vi "DisplayPanel.vi"() -> ()   [LabVIEW 2013]
uses:
  MvLVLib/MvCameraControl.lvlib
  <vilib>/picture/picture.llb/imagedata.ctl
panel:
  out "GenTLDevInfoArray":T1(array[cluster])
  out "GenTLIfInfoArray":T2(array[cluster])
  in  "Refresh Interaces":bool
  in  "Interface List":u16(ring)
  in  "pConvertInfo In":T3
  out "PixelFormat":u32
  out "handle out":u64
  in  "handle":u64
  in  "Rectangle":T4
  in  "image data":T5 caption="图像数据"
  out "Picture":picture
  out "PayloadSize":u32
  out "pFrameInfoEx out":T6
  out "nHeight":u32
  out "nWidth":u32
  out "Acquisision Flag":bool
  in  "Trigger Mode":bool
  in  "Continuous":bool
  out "打开标志":bool
  in  "stop":bool
  in  "Trigger Once":bool
  in  "Stop":bool
  in  "Start":bool
  in  "Open Device":bool
  in  "Close Device":bool
  in  "error in (no error) 2":errorcluster caption="错误输入（无错误）"
  in  "Refresh Devices":bool
  in  "Device List":u16(ring)
  # "Initialize"
  # "Acquisition"
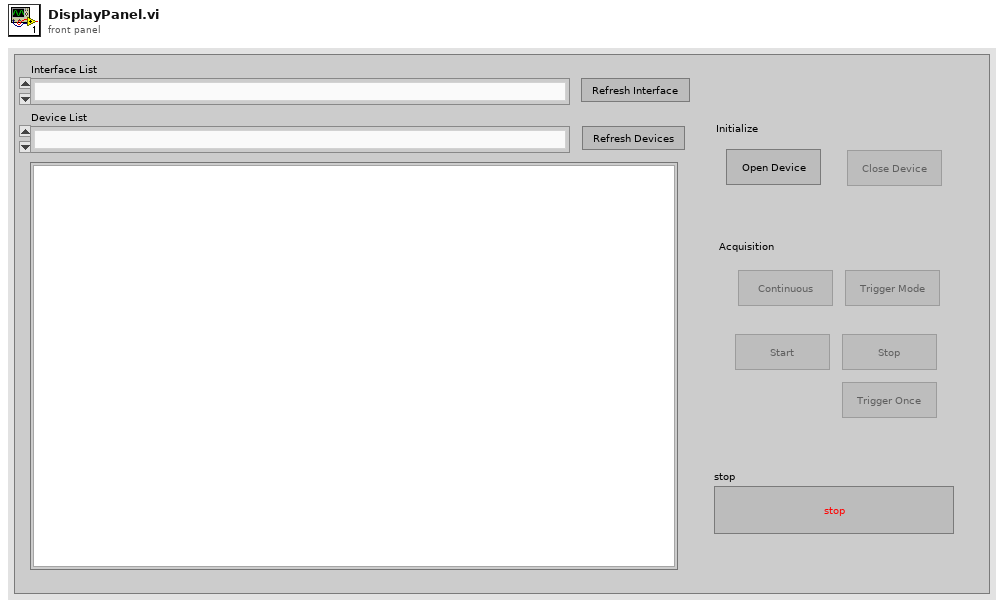
[diagram p1: front panel]
types:
  T1 = cluster{"chInterfaceID":string, "chDeviceID":string, "chVendorName":string, "chModelName":string, "chTLType":string, "chDisplayName":string, "chUserDefinedName":string, "chSerialNumber":string, "chDeviceVersion":string, "nCtiIndex":u32, "nReserved[0]":u32, "nReserved[1]":u32, "nReserved[2]":u32, "nReserved[3]":u32, "nReserved[4]":u32, "nReserved[5]":u32, "nReserved[6]":u32, "nReserved[7]":u32}[]
  T2 = cluster{"chInterfaceID":string, "chTLType":string, "chDisplayName":string, "nCtiIndex":u32, "nReserved[0]":u32, "nReserved[1]":u32, "nReserved[2]":u32, "nReserved[3]":u32, "nReserved[4]":u32, "nReserved[5]":u32, "nReserved[6]":u32, "nReserved[7]":u32}[]
  T3 = cluster{"nWidth":u16, "nHeight":u16, "enSrcPixelType":u32, "nSrcDataLen":u32, "enDstPixelType":u32, "nDstLen":u32, "nDstBufferSize":u32, "nRes0":u32, "nRes1":u32, "nRes2":u32, "nRes3":u32}
  T4 = cluster{"left":i16, "top":i16, "right":i16, "bottom":i16}
  T5 = typedef "imagedata.ctl" = cluster{"image type":i32, "image depth":i32, "image":u8[], "mask":u8[], "colors":u32[], "Rectangle":cluster{"left":i16, "top":i16, "right":i16, "bottom":i16}}
  T6 = cluster{"nWidth":u16, "nHeight":u16, "enPixelType":i32, "nFrameNum":u32, "nDevTimeStampHigh":u32, "nDevTimeStampLow":u32, "nReserved0":u32, "nHostTimeStamp":i64, "nFrameLen":u32, "nSecondCount]":u32, "nCycleCount":u32, "nCycleOffset":u32, "fGain":u32, "fExposureTime":u32, "nAverageBrightness":u32, "nRed":u32, "nGreen":u32, "nBlue":u32, "nFrameCounter":u32, "nTriggerIndex":u32, "nInput":u32, "nOutput":u32, "nOffsetX":u32, "nOffsetY":u32, "nReserved[0]":u32, "nReserved[1]":u32, "nReserved[2]":u32, "nReserved[3]":u32, "nReserved[4]":u32, "nReserved[5]":u32, "nReserved[6]":u32, "nReserved[7]":u32, "nReserved[8]":u32, "nReserved[9]":u32, "nReserved[10]":u32, "nReserved[11]":u32, "nReserved[12]":u32, "nReserved[13]":u32, "nReserved[14] 10":u32, "nReserved[15] 11":u32, "nReserved[16] 12":u32, "nReserved[17] 13":u32, "nReserved[18] 14":u32, "nReserved[19] 15":u32, "nReserved[20] 16":u32, "nReserved[21] 17":u32, "nReserved[22] 18":u32, "nReserved[23] 19":u32, "nReserved[24] 20":u32, "nReserved[25] 21":u32, "nReserved[26] 22":u32, "nReserved[27] 23":u32, "nReserved[28] 24":u32, "nReserved[29] 25":u32, "nReserved[30] 26":u32, "nReserved[31] 27":u32, "nReserved[32] 28":u32, "nReserved[33] 29":u32, "nReserved[34] 30":u32, "nReserved[35] 31":u32, "nReserved[36] 32":u32, "nReserved[37] 33":u32, "nReserved[38] 34":u32, "nReserved[39] 35":u32, "nReserved[40] 36":u32}
  T7 = enum8{"Enabled", "Disabled", "Disabled and Grayed Out"}
  T8 = cluster{"nCurValue":u32, "nMax":u32, "nMin":u32, "nInc":u32, "nReserved[0]":u32, "nReserved[1]":u32, "nReserved[2]":u32, "nReserved[3]":u32}
  T9 = cluster{"nCurValue":u32, "nSupportedNum":u32, "nSupportValue":u32[], "nReserved[0]":u32, "nReserved[1]":u32, "nReserved[2]":u32, "nReserved[3]":u32}
  T10 = cluster{"chInterfaceID":string, "chTLType":string, "chDisplayName":string, "nCtiIndex":u32, "nReserved[0]":u32, "nReserved[1]":u32, "nReserved[2]":u32, "nReserved[3]":u32, "nReserved[4]":u32, "nReserved[5]":u32, "nReserved[6]":u32, "nReserved[7]":u32}
  T11 = cluster{"nWidth":u32, "nHeight":u32, "enSrcPixelType":u32, "nSrcDataLen":u32, "enDstPixelType":u32, "nDstLen":u32, "nDstBufferSize":u32, "nRes0":u32, "nRes1":u32, "nRes2":u32, "nRes3":u32}
  T12 = cluster{"chInterfaceID":string, "chDeviceID":string, "chVendorName":string, "chModelName":string, "chTLType":string, "chDisplayName":string, "chUserDefinedName":string, "chSerialNumber":string, "chDeviceVersion":string, "nCtiIndex":u32, "nReserved[0]":u32, "nReserved[1]":u32, "nReserved[2]":u32, "nReserved[3]":u32, "nReserved[4]":u32, "nReserved[5]":u32, "nReserved[6]":u32, "nReserved[7]":u32}
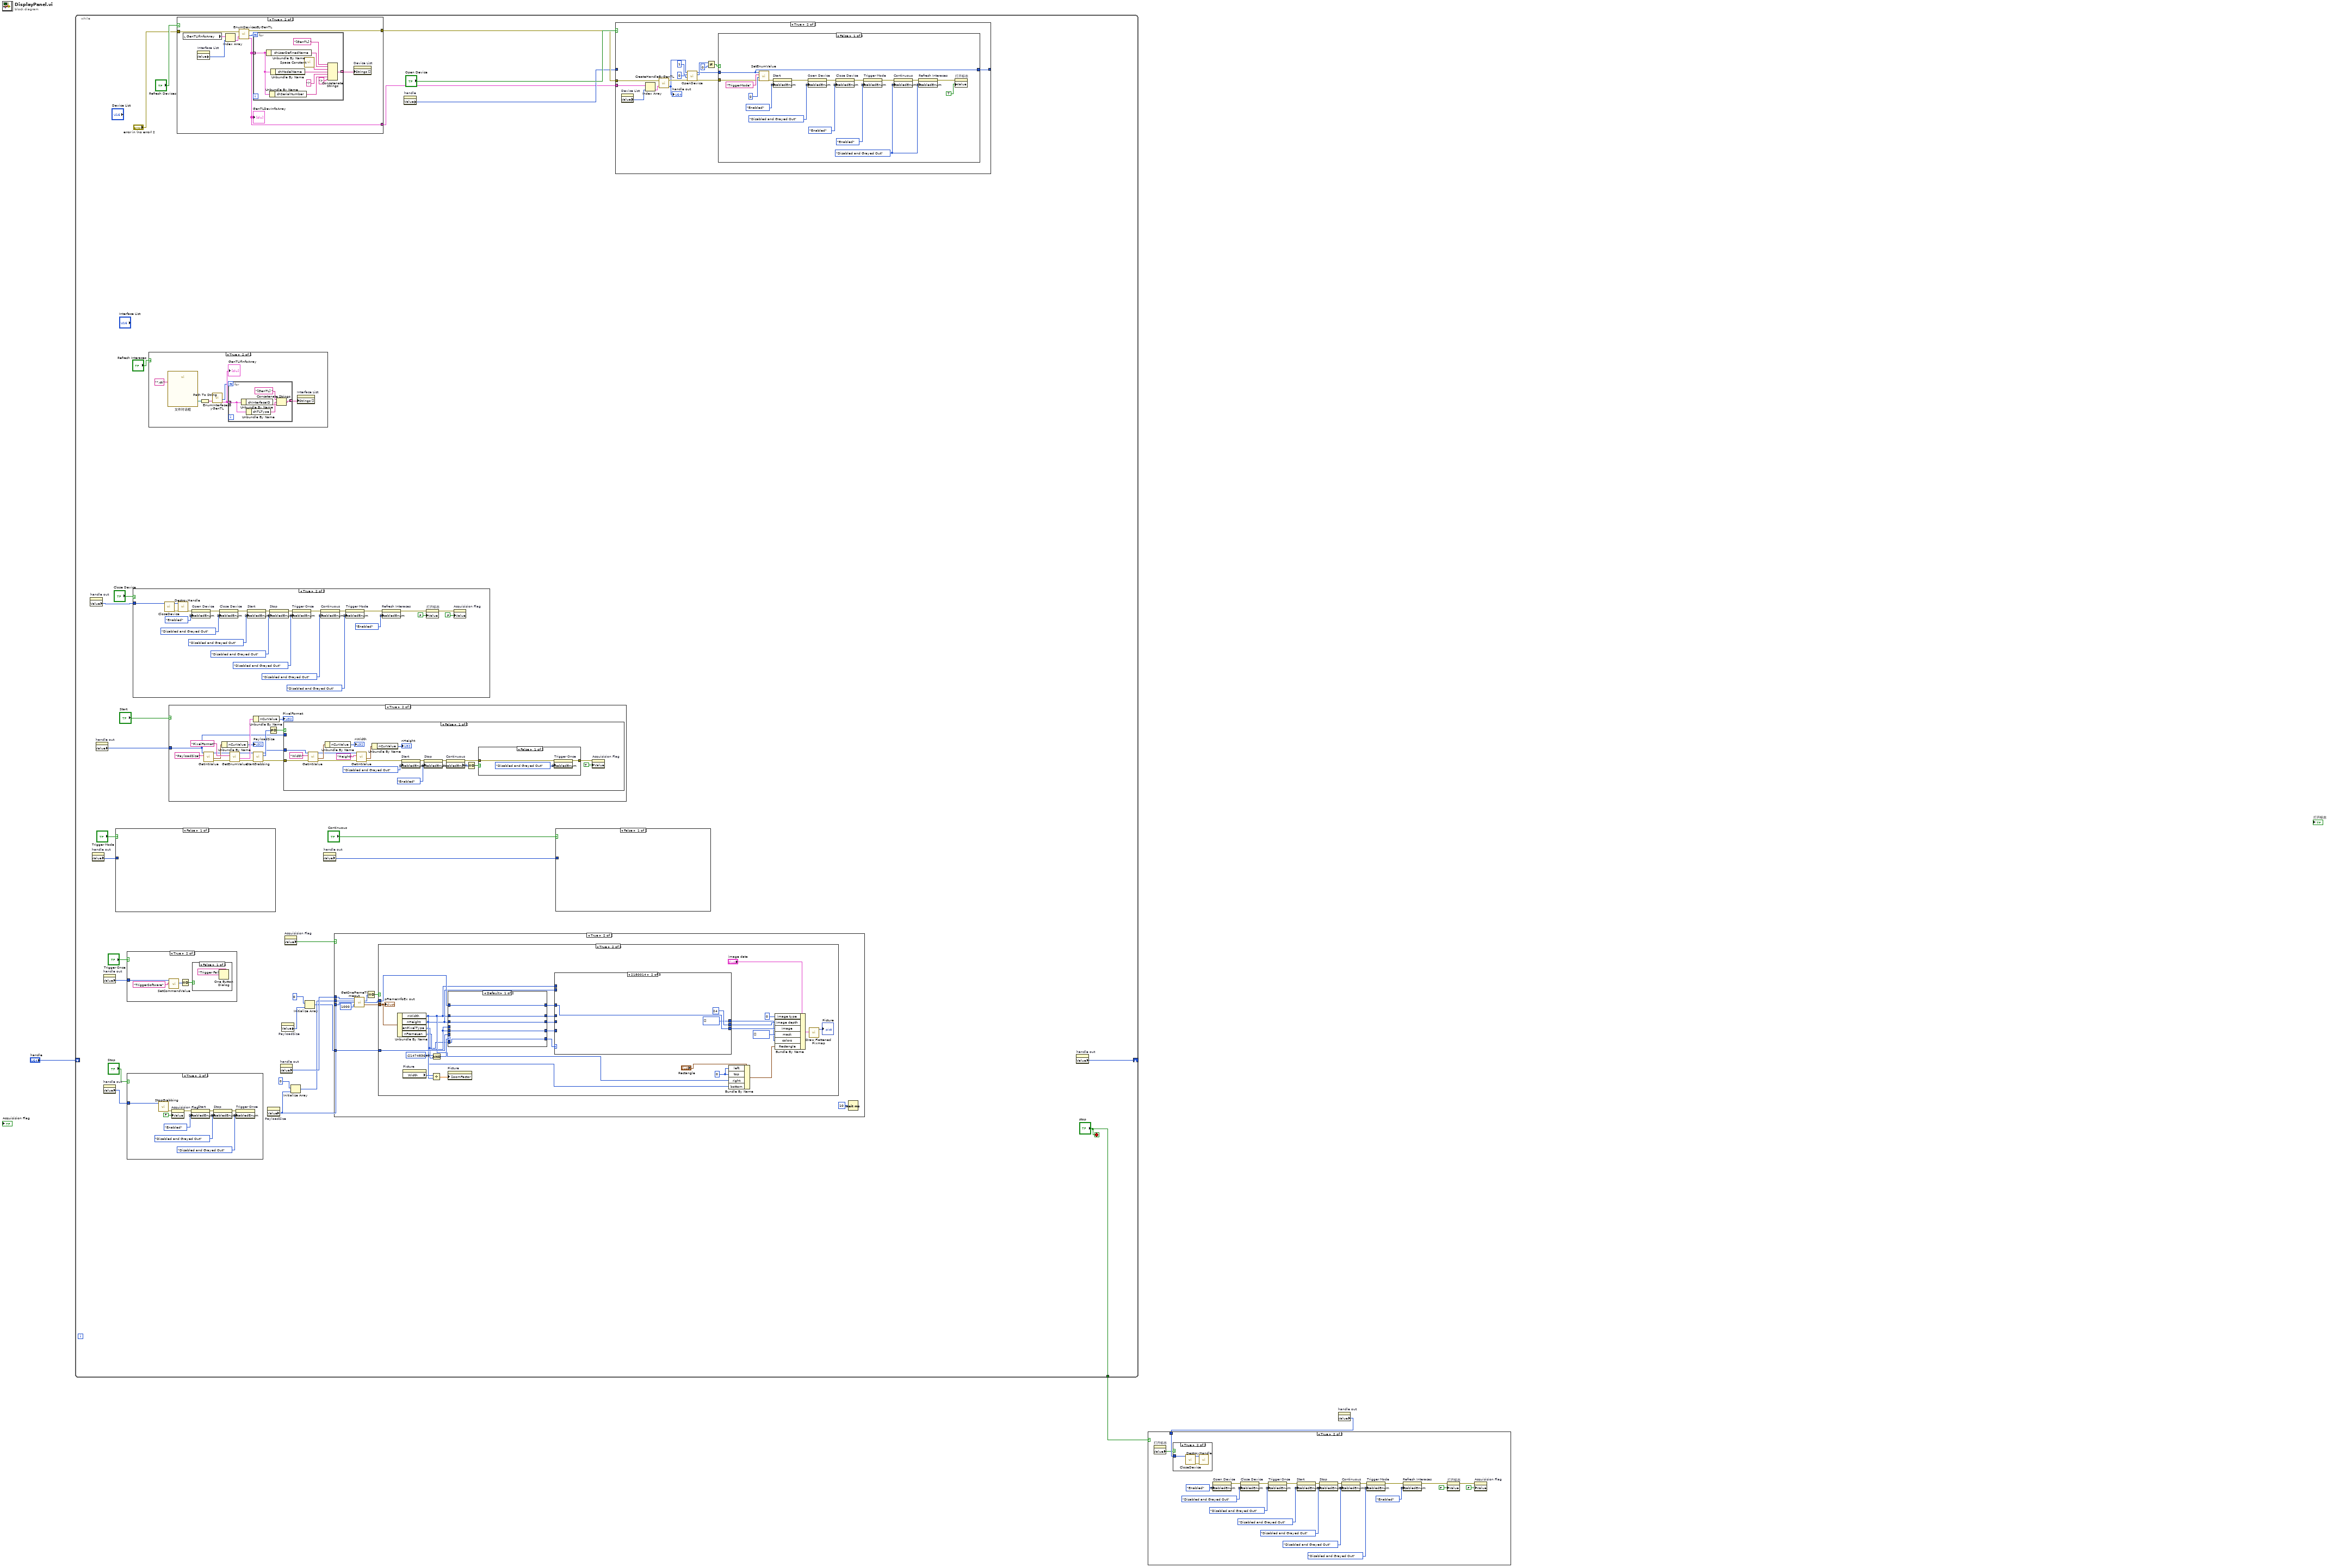
[diagram p0: block diagram]
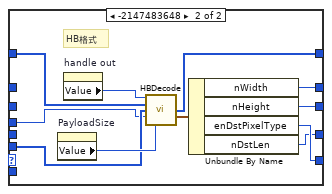
[diagram p7: hidden frame]
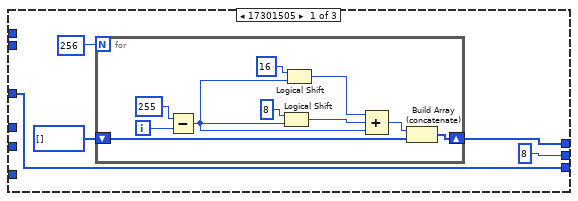
[diagram p8: hidden frame]
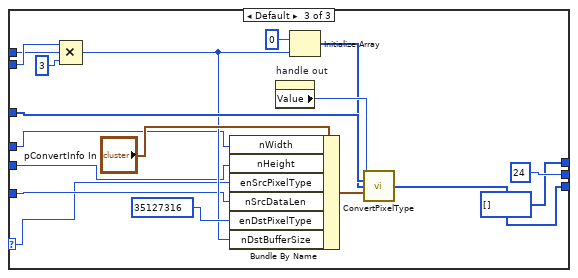
[diagram p9: hidden frame]
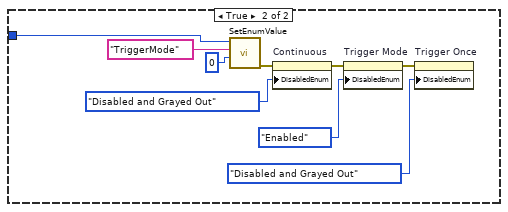
[diagram p11: hidden frame]
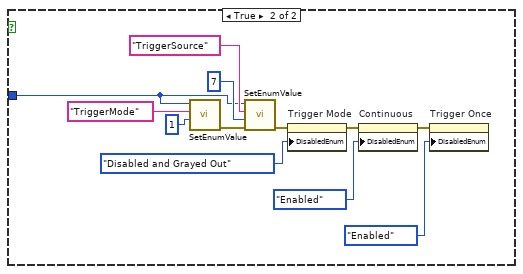
[diagram p12: hidden frame]
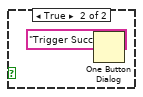
[diagram p14: hidden frame]
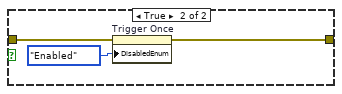
[diagram p16: hidden frame]
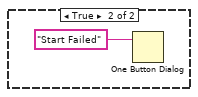
[diagram p17: hidden frame]
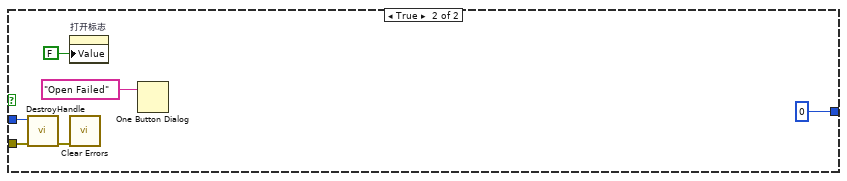
[diagram p20: hidden frame]
diagram:
  n1 = while {
    tunnel: ["stop"] -> w3
    shift-right: [w20] -> _
    shift-left: "handle" -> [_]
    stop <- "stop" stop-if-true
    n2 = property on="handle out" class="DigNum (strict)"() -> ("Value"=w18:u64)  [unwired: 2 in, 2 out]
    n3 = property on="handle out" class="DigNum (strict)"() -> ("Value"=w13:u64)  [unwired: 2 in, 2 out]
    n4 = property on="handle out" class="DigNum (strict)"() -> ("Value"=w14:u64)  [unwired: 2 in, 2 out]
    n5 = property on="handle out" class="DigNum (strict)"() -> ("Value"=w17:u64)  [unwired: 2 in, 2 out]
    n6 = property on="handle out" class="DigNum (strict)"() -> ("Value"=w16:u64)  [unwired: 2 in, 2 out]
    n7 = case shown="False" "Trigger Mode" {
      tunnel: w13 -> [_ w151]
      frame False {
      }
      frame True {
        n8 = call "SetEnumValue.vi"("nValue"=u32 1, "strKey"="TriggerMode", "handle"=w151) -> ("error out"=w157:errorcluster)  [unwired: 6 in, 2 out]
        n9 = call "SetEnumValue.vi"("error in (no error)"=w157, "nValue"=u32 7, "strKey"="TriggerSource", "handle"=w151) -> ("error out"=w156:errorcluster)  [unwired: 5 in, 2 out]
        n10 = property on="Trigger Mode" class="Bool"(error in=w156, "DisabledEnum"=T7."Disabled and Grayed Out" ("禁用")) -> (error out=w155:errorcluster)  [unwired: 1 in, 1 out]
        n11 = property on="Continuous" class="Bool"(error in=w155, "DisabledEnum"=T7."Enabled" ("禁用")) -> (error out=w153:errorcluster)  [unwired: 1 in, 1 out]
        n12 = property on="Trigger Once" class="Bool"(error in=w153, "DisabledEnum"=T7."Enabled" ("禁用")) -> ()  [unwired: 1 in, 2 out]
      }
    }
    n13 = case shown="True" "Trigger Once" {
      tunnel: w17 -> [_ w166]
      frame False {
      }
      frame True {
        n14 = call "SetCommandValue.vi"("strValue"="TriggerSoftware", "handle"=w166) -> ("function return"=w164:i32)  [unwired: 7 in, 2 out]
        n15 = Equal To 0?(x=w164) -> (x = 0?=w163:bool)
        n16 = case shown="False" w163 {
          frame False {
            n17 = One Button Dialog(message="Trigger Failed") -> ()  [unwired: 1 in, 1 out]
          }
          frame True {
            n18 = One Button Dialog(message="Trigger Success") -> ()  [unwired: 1 in, 1 out]
          }
        }
      }
    }
    n19 = case shown="True" "Stop" {
      tunnel: w16 -> [_ w141]
      frame False {
      }
      frame True {
        n20 = call "StopGrabbing.vi"("handle"=w141) -> ("error out"=w140:errorcluster)  [unwired: 8 in, 2 out]
        n21 = property on="Acquisision Flag" class="Bool (strict)"(error in=w140, "Value"=FALSE ("采集标志")) -> (error out=w135:errorcluster)  [unwired: 1 in, 1 out]
        n22 = property on="Start" class="Bool"(error in=w135, "DisabledEnum"=T7."Enabled" ("禁用")) -> (error out=w134:errorcluster)  [unwired: 1 in, 1 out]
        n23 = property on="Stop" class="Bool"(error in=w134, "DisabledEnum"=T7."Disabled and Grayed Out" ("禁用")) -> (error out=w133:errorcluster)  [unwired: 1 in, 1 out]
        n24 = property on="Trigger Once" class="Bool"(error in=w133, "DisabledEnum"=T7."Disabled and Grayed Out" ("禁用")) -> ()  [unwired: 1 in, 2 out]
      }
    }
    n25 = case shown="True" "Close Device" {
      tunnel: w18 -> [_ w216]
      frame False {
      }
      frame True {
        n26 = call "CloseDevice.vi"("handle"=w216) -> ("error out"=w218:errorcluster, "handle out"=w215:u64)  [unwired: 8 in, 1 out]
        n27 = call "DestroyHandle.vi"("error in (no error)"=w218, "handle"=w215) -> ("error out"=w217:errorcluster)  [unwired: 8 in, 1 out]
        n28 = property on="Open Device" class="Bool"(error in=w217, "DisabledEnum"=T7."Enabled" ("禁用")) -> (error out=w229:errorcluster)  [unwired: 1 in, 1 out]
        n29 = property on="Close Device" class="Bool"(error in=w229, "DisabledEnum"=T7."Disabled and Grayed Out" ("禁用")) -> (error out=w228:errorcluster)  [unwired: 1 in, 1 out]
        n30 = property on="Start" class="Bool"(error in=w228, "DisabledEnum"=T7."Disabled and Grayed Out" ("禁用")) -> (error out=w227:errorcluster)  [unwired: 1 in, 1 out]
        n31 = property on="Stop" class="Bool"(error in=w227, "DisabledEnum"=T7."Disabled and Grayed Out" ("禁用")) -> (error out=w226:errorcluster)  [unwired: 1 in, 1 out]
        n32 = property on="Trigger Once" class="Bool"(error in=w226, "DisabledEnum"=T7."Disabled and Grayed Out" ("禁用")) -> (error out=w223:errorcluster)  [unwired: 1 in, 1 out]
        n33 = property on="Continuous" class="Bool"(error in=w223, "DisabledEnum"=T7."Disabled and Grayed Out" ("禁用")) -> (error out=w222:errorcluster)  [unwired: 1 in, 1 out]
        n34 = property on="Trigger Mode" class="Bool"(error in=w222, "DisabledEnum"=T7."Disabled and Grayed Out" ("禁用")) -> (error out=w213:errorcluster)  [unwired: 1 in, 1 out]
        n35 = property on="Refresh Interaces" class="Bool"(error in=w213, "DisabledEnum"=T7."Enabled" ("禁用")) -> (error out=w212:errorcluster)  [unwired: 1 in, 1 out]
        n36 = property on="打开标志" class="Bool (strict)"(error in=w212, "Value"=FALSE ("打开标志")) -> (error out=w220:errorcluster)  [unwired: 1 in, 1 out]
        n37 = property on="Acquisision Flag" class="Bool (strict)"(error in=w220, "Value"=FALSE ("采集标志")) -> ()  [unwired: 1 in, 2 out]
      }
    }
    n38 = case shown="True" "Refresh Interaces" {
      frame False {
      }
      frame True {
        n39 = call "文件对话框"("pattern (all files)"="*.cti") -> ("selected path"=w37:path)  [unwired: 11 in, 3 out]
        n40 = Path To String(path=w37) -> (string=w36:string)
        n41 = call "EnumInterfacesByGenTL.vi"("strGenTLPath"=w36) -> ("nInterfaceNum"=w34:u32, "pGenTLIfInfoArray"=w35:T2)  [unwired: 1 in, 2 out]
        "GenTLIfInfoArray" <- w35
        n42 = for {
          N: w34 -> [_]
          tunnel: [w43] -> w33 mode=indexing
          tunnel: w35 -> [w40] mode=indexing
          n43 = Unbundle By Name(w40) -> ("chInterfaceID"=w41:string)
          n44 = Unbundle By Name(w40) -> ("chTLType"=w39:string)
          n45 = Concatenate Strings("[GenTL] " ("字符串"), w39, w41) -> (w43:string)
        }
        n46 = property on="Interface List" class="Ring (strict)"("Strings []"=w33) -> ()  [unwired: 2 in, 2 out]
      }
    }
    n47 = case shown="True" "Start" {
      tunnel: w14 -> [_ w173]
      frame False {
      }
      frame True {
        n48 = call "GetIntValue.vi"("strKey"="PayloadSize", "handle"=w173) -> ("error out"=w179:errorcluster, "pIntValue out"=w175:T8, "handle out"=w171:u64)  [unwired: 6 in, 1 out]
        n49 = Unbundle By Name(w175) -> ("nCurValue"=→"PayloadSize":u32)
        n50 = call "GetEnumValue.vi"("error in (no error)"=w179, "strKey"="PixelFormat", "handle"=w171) -> ("error out"=w178:errorcluster, "pEnumValue out"=w180:T9, "handle out"=w170:u64)  [unwired: 5 in, 1 out]
        n51 = Unbundle By Name(w180) -> ("nCurValue"=→"PixelFormat":u32)
        n52 = call "StartGrabbing.vi"("error in (no error)"=w178, "handle"=w170) -> ("error out"=w177:errorcluster, "function return"=w183:i32, "handle out"=w169:u64)  [unwired: 7 in]
        n53 = Not Equal To 0?(x=w183) -> (x != 0?=w182:bool)
        n54 = case shown="False" w182 {
          tunnel: w173 -> [_ _]
          tunnel: w177 -> [w186 _]
          tunnel: w169 -> [w185 _]
          frame False {
            n55 = call "GetIntValue.vi"("error in (no error)"=w186, "strKey"="Width", "handle"=w185) -> ("error out"=w193:errorcluster, "pIntValue out"=w187:T8, "handle out"=w184:u64)  [unwired: 5 in, 1 out]
            n56 = Unbundle By Name(w187) -> ("nCurValue"=→"nWidth":u32)
            n57 = call "GetIntValue.vi"("error in (no error)"=w193, "strKey"="Height", "handle"=w184) -> ("error out"=w192:errorcluster, "pIntValue out"=w190:T8)  [unwired: 5 in, 2 out]
            n58 = Unbundle By Name(w190) -> ("nCurValue"=→"nHeight":u32)
            n59 = property on="Start" class="Bool"(error in=w192, "DisabledEnum"=T7."Disabled and Grayed Out" ("禁用")) -> (error out=w202:errorcluster)  [unwired: 1 in, 1 out]
            n60 = property on="Stop" class="Bool"(error in=w202, "DisabledEnum"=T7."Enabled" ("禁用")) -> (error out=w188:errorcluster)  [unwired: 1 in, 1 out]
            n61 = property on="Continuous" class="Bool"(error in=w188) -> (error out=w198:errorcluster, "DisabledEnum"=w199:T7)  [unwired: 1 in, 1 out]
            n62 = Equal To 0?(x=w199) -> (x = 0?=w200:bool)
            n63 = case shown="False" w200 {
              tunnel: w198 -> [w205 w208]
              tunnel: [w204 w207] -> w197
              frame False {
                n64 = property on="Trigger Once" class="Bool"(error in=w205, "DisabledEnum"=T7."Disabled and Grayed Out" ("禁用")) -> (error out=w204:errorcluster)  [unwired: 1 in, 1 out]
              }
              frame True {
                n65 = property on="Trigger Once" class="Bool"(error in=w208, "DisabledEnum"=T7."Enabled" ("禁用")) -> (error out=w207:errorcluster)  [unwired: 1 in, 1 out]
              }
            }
            n66 = property on="Acquisision Flag" class="Bool (strict)"(error in=w197, "Value"=TRUE ("采集标志")) -> ()  [unwired: 1 in, 2 out]
          }
          frame True {
            n67 = One Button Dialog(message="Start Failed") -> ()  [unwired: 1 in, 1 out]
          }
        }
      }
    }
    n68 = case shown="True" "Refresh Devices" {
      tunnel: [w273 w276] -> w22
      tunnel: "error in (no error) 2" -> [w273 w277]
      tunnel: [w272 w274] -> w7
      frame False {
        n69 = local read "GenTLDevInfoArray"() -> (w272:T1)
      }
      frame True {
        n70 = local read "GenTLIfInfoArray"() -> (w279:T2)
        n71 = property on="Interface List" class="Ring (strict)"() -> ("Value"=w280:u16)  [unwired: 2 in, 2 out]
        n72 = Index Array(array=w279, index=w280) -> (element=w278:T10)
        n73 = call "EnumDevicesByGenTL.vi"("error in (no error)"=w277, "pIFInfo"=w278) -> ("error out"=w276:errorcluster, "nDeviceNum"=w275:u32, "pGenTLDevInfoArray"=w274:T1)  [unwired: 1 out]
        "GenTLDevInfoArray" <- w274
        n74 = for {
          N: w275 -> [_]
          tunnel: [w287] -> w281 mode=indexing
          tunnel: w274 -> [w285] mode=indexing
          n75 = Unbundle By Name(w285) -> ("chUserDefinedName"=w284:string)
          n76 = Unbundle By Name(w285) -> ("chSerialNumber"=w282:string)
          n77 = Unbundle By Name(w285) -> ("chModelName"=w283:string)
          n78 = call <vilib>:"Space Constant.vi"() -> ("String"=w290:string)
          n79 = Concatenate Strings("[GenTL] " ("字符串"), w284, w290, w283, "(" ("字符串"), w282, ")" ("字符串")) -> (w287:string)
        }
        n80 = property on="Device List" class="Ring (strict)"("Strings []"=w281) -> ()  [unwired: 2 in, 2 out]
      }
    }
    n81 = property on="PayloadSize" class="DigNum (strict)"() -> ("Value"=w9:u32)  [unwired: 2 in, 2 out]
    n82 = property on="handle out" class="DigNum (strict)"() -> ("Value"=w15:u64)  [unwired: 2 in, 2 out]
    n83 = property on="PayloadSize" class="DigNum (strict)"() -> ("Value"=w6:u32)  [unwired: 2 in, 2 out]
    n84 = property on="Acquisision Flag" class="Bool (strict)"() -> ("Value"=w24:bool)  [unwired: 2 in, 2 out]
    n85 = Initialize Array(u8 0 ("元素"), w9) -> (w10:u8[])
    n86 = Initialize Array(u8 0 ("元素"), w6) -> (w5:u8[])
    n87 = property on="handle out" class="DigNum (strict)"() -> ("Value"=w12:u64)  [unwired: 2 in, 2 out]
    n88 = case shown="True" w24 {
      tunnel: w15 -> [_ w50]
      tunnel: w10 -> [_ w49]
      tunnel: w9 -> [_ w48]
      tunnel: w5 -> [_ w44]
      frame False {
      }
      frame True {
        n89 = call "GetOneFrameTimeout.vi"("handle"=w50, "pData"=w49, "nDataSize"=w48, "nMsec"=1000) -> ("function return"=w47:i32, "pData Out"=w46:u8[], "pFrameInfoEx out"=w45:T6)  [unwired: 7 in, 2 out]
        n90 = Equal To 0?(x=w47) -> (x = 0?=w52:bool)
        n91 = case shown="True" w52 {
          tunnel: w46 -> [_ w63]
          tunnel: w45 -> [_ w67]
          tunnel: w44 -> [_ w64]
          frame False {
          }
          frame True {
            w77 = i16 0 ("left")
            n92 = Unbundle By Name(w67) -> ("nWidth"=w62:u16, "nHeight"=w61:u16, "enPixelType"=w54:i32, "nFrameLen"=w60:u32)
            n93 = property on="Picture" class="Pict"() -> ("Width"=w72:u32)  [unwired: 2 in, 2 out]
            n94 = Divide(x=w72, y=w62) -> (x/y=w71:dbl)
            n95 = Compound Arithmetic op=AND(-2147483648 ("value"), w54) -> (w65:i32)
            n96 = case shown="Default" w65 {
              tunnel: [w85 w93] -> w59
              tunnel: [w84 w92] -> w58
              tunnel: [w83 w91] -> w57
              tunnel: [w81 w90] -> w55
              tunnel: [w82 w89] -> w56
              tunnel: w64 -> [_ w88]
              tunnel: w63 -> [w85 w87]
              tunnel: w60 -> [_ w86]
              tunnel: w62 -> [w84 _]
              tunnel: w61 -> [w83 _]
              tunnel: w60 -> [w82 _]
              tunnel: w54 -> [w81 _]
              frame Default {
              }
              frame -2147483648 {
                # "HB格式"
                n97 = property on="PayloadSize" class="DigNum (strict)"() -> ("Value"=w95:u32)  [unwired: 2 in, 2 out]
                n98 = property on="handle out" class="DigNum (strict)"() -> ("Value"=w96:u64)  [unwired: 2 in, 2 out]
                n99 = call "HBDecode.vi"("handle"=w96, "pSrcData"=w87, "pDstBuf In"=w88, "SrcDataLen"=w86, "DstBufferSize"=w95) -> ("pDstBuf Out"=w93:u8[], "pHBDecode Out"=w94:T11)  [unwired: 6 in, 3 out]
                n100 = Unbundle By Name(w94) -> ("nWidth"=w92:u32, "nHeight"=w91:u32, "enDstPixelType"=w90:u32, "nDstLen"=w89:u32)
              }
            }
            n101 = property on="Picture" class="Pict"("ZoomFactor"=w71) -> ()  [unwired: 2 in, 2 out]
            n102 = case shown="2180014" w55 {
              selector: w55 -> [_ _ w115]
              tunnel: w59 -> [w99 w114 w129]
              tunnel: w61 -> [_ _ w126]
              tunnel: w62 -> [_ _ w125]
              tunnel: [w99 w114 w119] -> w70
              tunnel: [8 24 24] -> w69
              tunnel: [w97 i32[] [] i32[] []] -> w68
              tunnel: w58 -> [_ _ w118]
              tunnel: w57 -> [_ _ w117]
              tunnel: w56 -> [_ _ w116]
              frame 17301505 {
                n103 = for {
                  N: 256 -> [_]
                  shift-right: [w106] -> w97
                  shift-left: i32[] [] ("数组") -> [w105]
                  i -> [w102]
                  n104 = Subtract(x=255, y=w102) -> (x-y=w103:i32)
                  n105 = Logical Shift(y=i16 8, x=w103) -> (x << y=w108:i32)
                  n106 = Logical Shift(y=16 ("x"), x=w103) -> (x << y=w109:i32)
                  n107 = Compound Arithmetic op=ADD(w109, w108, w103) -> (w107:i32)
                  n108 = Build Array (concatenate)(w107, w105) -> (w106:i32[])
                }
              }
              frame 35127316 {
              }
              frame Default {
                n109 = Compound Arithmetic op=MULTIPLY(w126, w125, u32 3 ("值")) -> (w123:u32)
                n110 = Bundle By Name(cluster="pConvertInfo In", "nWidth"=w118, "nHeight"=w117, "enSrcPixelType"=w115, "nSrcDataLen"=w116, "enDstPixelType"=u32 35127316, "nDstBufferSize"=w123) -> (w122:T3)
                n111 = property on="handle out" class="DigNum (strict)"() -> ("Value"=w130:u64)  [unwired: 2 in, 2 out]
                n112 = Initialize Array(u8 0 ("元素"), w123) -> (w128:u8[])
                n113 = call "ConvertPixelType.vi"("handle"=w130, "pSrcData"=w129, "pDstBuf In"=w128, "pConvertInfo In"=w122) -> ("pDstBuf Out"=w119:u8[])  [unwired: 7 in, 4 out]
              }
            }
            n114 = Bundle By Name(cluster="Rectangle", "left"=w77, "top"=w77, "right"=w62, "bottom"=w61) -> (w74:T4)
            n115 = Bundle By Name(cluster="image data", "image type"=0, "image depth"=w69, "image"=w70, "mask"=u8[] [], "colors"=w68, "Rectangle"=w74) -> (w73:T5)
            n116 = call <vilib>:"Draw Flattened Pixmap.vi"("image data"=w73) -> ("new picture"=→"Picture":picture)  [unwired: 8 in]
            "pFrameInfoEx out" <- w67
          }
        }
        n117 = Wait (ms)(milliseconds to wait=u32 10 ("等待时间（毫秒）")) -> ()  [unwired: 1 out]
      }
    }
    n118 = property on="handle" class="DigNum (strict)"() -> ("Value"=w19:u64)  [unwired: 2 in, 2 out]
    n119 = case shown="False" "Continuous" {
      tunnel: w12 -> [_ w142]
      frame False {
      }
      frame True {
        n120 = call "SetEnumValue.vi"("nValue"=u32 0, "strKey"="TriggerMode", "handle"=w142) -> ("error out"=w143:errorcluster)  [unwired: 6 in, 2 out]
        n121 = property on="Continuous" class="Bool"(error in=w143, "DisabledEnum"=T7."Disabled and Grayed Out" ("禁用")) -> (error out=w147:errorcluster)  [unwired: 1 in, 1 out]
        n122 = property on="Trigger Mode" class="Bool"(error in=w147, "DisabledEnum"=T7."Enabled" ("禁用")) -> (error out=w145:errorcluster)  [unwired: 1 in, 1 out]
        n123 = property on="Trigger Once" class="Bool"(error in=w145, "DisabledEnum"=T7."Disabled and Grayed Out" ("禁用")) -> ()  [unwired: 1 in, 2 out]
      }
    }
    n124 = case shown="True" "Open Device" {
      tunnel: [w234 w243] -> _
      tunnel: w19 -> [w234 _]
      tunnel: w22 -> [_ w238]
      tunnel: w7 -> [_ w236]
      frame False {
      }
      frame True {
        n125 = property on="Device List" class="Ring (strict)"() -> ("Value"=w240:u16)  [unwired: 2 in, 2 out]
        n126 = Index Array(array=w236, index=w240) -> (element=w235:T12)
        n127 = call "CreateHandleByGenTL.vi"("error in (no error)"=w238, "pDevInfo"=w235) -> ("error out"=w239:errorcluster, "handle"=w237:u64)  [unwired: 1 out]
        "handle out" <- w237
        n128 = call "OpenDevice.vi"("error in (no error)"=w239, "nSwitchoverKey"=u16 0, "nAccessMode"=u32 1, "handle"=w237) -> ("error out"=w244:errorcluster, "return"=w242:i32, "handle out"=w241:u64)  [unwired: 5 in]
        n129 = Not Equal?(x=w242, y=0) -> (x != y?=w247:bool)
        n130 = case shown="False" w247 {
          tunnel: w241 -> [w252 w269]
          tunnel: w244 -> [w253 w266]
          tunnel: [w252 u64 0 ("handle")] -> w243
          frame False {
            w251 = T7."Disabled and Grayed Out" ("禁用")
            n131 = call "SetEnumValue.vi"("error in (no error)"=w253, "nValue"=u32 0, "strKey"="TriggerMode", "handle"=w252) -> ("error out"=w262:errorcluster)  [unwired: 5 in, 2 out]
            n132 = property on="Start" class="Bool"(error in=w262, "DisabledEnum"=T7."Enabled" ("禁用")) -> (error out=w260:errorcluster)  [unwired: 1 in, 1 out]
            n133 = property on="Open Device" class="Bool"(error in=w260, "DisabledEnum"=T7."Disabled and Grayed Out" ("禁用")) -> (error out=w259:errorcluster)  [unwired: 1 in, 1 out]
            n134 = property on="Close Device" class="Bool"(error in=w259, "DisabledEnum"=T7."Enabled" ("禁用")) -> (error out=w256:errorcluster)  [unwired: 1 in, 1 out]
            n135 = property on="Trigger Mode" class="Bool"(error in=w256, "DisabledEnum"=T7."Enabled" ("禁用")) -> (error out=w255:errorcluster)  [unwired: 1 in, 1 out]
            n136 = property on="Continuous" class="Bool"(error in=w255, "DisabledEnum"=w251) -> (error out=w250:errorcluster)  [unwired: 1 in, 1 out]
            n137 = property on="Refresh Interaces" class="Bool"(error in=w250, "DisabledEnum"=w251) -> (error out=w249:errorcluster)  [unwired: 1 in, 1 out]
            n138 = property on="打开标志" class="Bool (strict)"(error in=w249, "Value"=TRUE ("布尔")) -> ()  [unwired: 1 in, 2 out]
          }
          frame True {
            n139 = call "DestroyHandle.vi"("error in (no error)"=w266, "handle"=w269) -> ("error out"=w267:errorcluster)  [unwired: 8 in, 1 out]
            n140 = property on="打开标志" class="Bool (strict)"("Value"=FALSE) -> ()  [unwired: 2 in, 2 out]
            n141 = call <vilib>:"Clear Errors.vi"("error in (no error)"=w267) -> ()  [unwired: 5 in, 2 out]
            n142 = One Button Dialog(message="Open Failed") -> ()  [unwired: 1 in, 1 out]
          }
        }
      }
    }
    n143 = property on="handle out" class="DigNum (strict)"() -> ("Value"=w20:u64)  [unwired: 2 in, 2 out]
  }
  n144 = property on="handle out" class="DigNum (strict)"() -> ("Value"=w1:u64)  [unwired: 2 in, 2 out]
  n145 = case shown="True" w3 {
    tunnel: w1 -> [_ w306]
    frame False {
    }
    frame True {
      n146 = property on="打开标志" class="Bool (strict)"() -> ("Value"=w297:bool)  [unwired: 2 in, 2 out]
      n147 = case shown="True" w297 {
        tunnel: w306 -> [_ w313]
        frame False {
        }
        frame True {
          n148 = call "CloseDevice.vi"("handle"=w313) -> ("error out"=w314:errorcluster, "handle out"=w312:u64)  [unwired: 8 in, 1 out]
          n149 = call "DestroyHandle.vi"("error in (no error)"=w314, "handle"=w312) -> ()  [unwired: 8 in, 2 out]
        }
      }
      n150 = property on="Open Device" class="Bool"("DisabledEnum"=T7."Enabled" ("禁用")) -> (error out=w305:errorcluster)  [unwired: 2 in, 1 out]
      n151 = property on="Close Device" class="Bool"(error in=w305, "DisabledEnum"=T7."Disabled and Grayed Out" ("禁用")) -> (error out=w304:errorcluster)  [unwired: 1 in, 1 out]
      n152 = property on="Trigger Once" class="Bool"(error in=w304, "DisabledEnum"=T7."Disabled and Grayed Out" ("禁用")) -> (error out=w303:errorcluster)  [unwired: 1 in, 1 out]
      n153 = property on="Start" class="Bool"(error in=w303, "DisabledEnum"=T7."Disabled and Grayed Out" ("禁用")) -> (error out=w302:errorcluster)  [unwired: 1 in, 1 out]
      n154 = property on="Stop" class="Bool"(error in=w302, "DisabledEnum"=T7."Disabled and Grayed Out" ("禁用")) -> (error out=w301:errorcluster)  [unwired: 1 in, 1 out]
      n155 = property on="Continuous" class="Bool"(error in=w301, "DisabledEnum"=T7."Disabled and Grayed Out" ("禁用")) -> (error out=w299:errorcluster)  [unwired: 1 in, 1 out]
      n156 = property on="Trigger Mode" class="Bool"(error in=w299, "DisabledEnum"=T7."Disabled and Grayed Out" ("禁用")) -> (error out=w292:errorcluster)  [unwired: 1 in, 1 out]
      n157 = property on="Refresh Interaces" class="Bool"(error in=w292, "DisabledEnum"=T7."Enabled" ("禁用")) -> (error out=w291:errorcluster)  [unwired: 1 in, 1 out]
      n158 = property on="打开标志" class="Bool (strict)"(error in=w291, "Value"=FALSE ("打开标志")) -> (error out=w294:errorcluster)  [unwired: 1 in, 1 out]
      n159 = property on="Acquisision Flag" class="Bool (strict)"(error in=w294, "Value"=FALSE ("采集标志")) -> ()  [unwired: 1 in, 2 out]
    }
  }
